vi "INST_PS_MEAS_2.0.0.vi"(4 "Use OPC?(T)":bool=TRUE, 6 "Instrument Select (Output 1)":string(combo)="1", 7 "Clear Error in":bool, 8 "error in (no error)":errorcluster, 9 "Measurement Type (Voltage)":string(combo)="MEAS:VOLT?", 11 "VISA session":refnum<visa-resource-name>) -> (0 "error out":errorcluster, 1 "Measurement (str)":string, 2 "Measurement":dbl format="%.2p", 3 "dup VISA session":refnum<visa-resource-name>)   [LabVIEW 2018]
doc: "This VI takes a measurement on the output signal and returns the measured value."
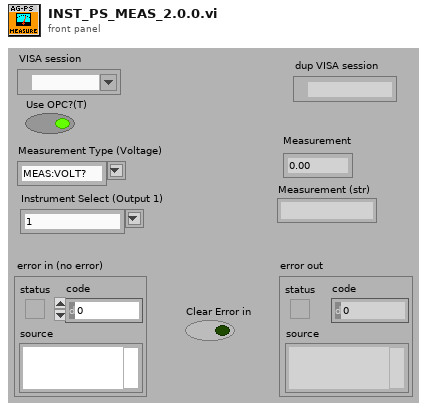
[diagram p1: front panel]
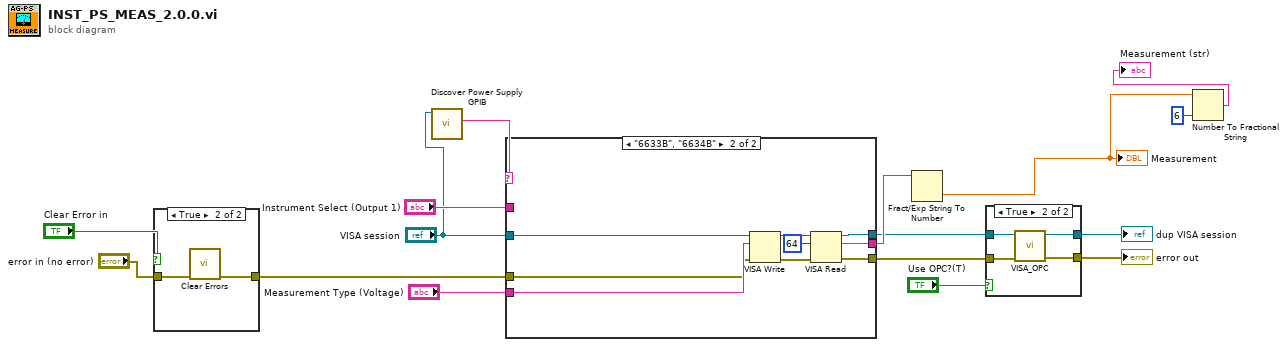
[diagram p0: block diagram]
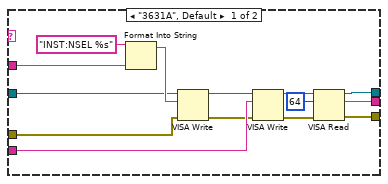
[diagram p2: hidden frame]
diagram:
  n1 = case shown="True" "Clear Error in" {
    tunnel: "error in (no error)" -> [w17 w19]
    tunnel: [w17 w18] -> w7
    frame False {
    }
    frame True {
      n2 = call <vilib>:"Clear Errors.vi"("error in (no error)"=w19) -> ("error out"=w18:errorcluster)  [unwired: 5 in, 1 out]
    }
  }
  n3 = call "Discover Power Supply GPIB.vi"("ADDRESS IN"="VISA session") -> ("PSn Model"=w5:string)  [unwired: 10 in]
  n4 = case shown="\"6633B\", \"6634B\"" w5 {
    tunnel: [w31 w40] -> w16
    tunnel: "Measurement Type (Voltage)" -> [w29 w38]
    tunnel: "Instrument Select (Output 1)" -> [w28 _]
    tunnel: "VISA session" -> [w23 w35]
    tunnel: [w22 w37] -> w13
    tunnel: [w21 w36] -> w10
    tunnel: w7 -> [w20 w34]
    frame "3631A", Default {
      n5 = Format Into String(format string="INST:NSEL %s", w28) -> (resulting string=w26:string)  [unwired: 2 in, 1 out]
      n6 = VISA Write(VISA resource name=w23, write buffer=w26, error in (no error)=w20) -> (VISA resource name out=w24:refnum<visa-resource-name>, error out=w25:errorcluster)  [unwired: 1 out]
      n7 = VISA Write(VISA resource name=w24, write buffer=w29, error in (no error)=w25) -> (VISA resource name out=w30:refnum<visa-resource-name>, error out=w33:errorcluster)  [unwired: 1 out]
      n8 = VISA Read(VISA resource name=w30, byte count=u32 64, error in (no error)=w33) -> (VISA resource name out=w21:refnum<visa-resource-name>, read buffer=w31:string, error out=w22:errorcluster)  [unwired: 1 out]
    }
    frame "6633B", "6634B" {
      n9 = VISA Write(VISA resource name=w35, write buffer=w38, error in (no error)=w34) -> (VISA resource name out=w39:refnum<visa-resource-name>, error out=w42:errorcluster)  [unwired: 1 out]
      n10 = VISA Read(VISA resource name=w39, byte count=u32 64, error in (no error)=w42) -> (VISA resource name out=w36:refnum<visa-resource-name>, read buffer=w40:string, error out=w37:errorcluster)  [unwired: 1 out]
    }
  }
  n11 = Fract/Exp String To Number(string=w16) -> (number=w3:dbl)  [unwired: 3 in, 1 out]
  "Measurement" <- w3
  n12 = case shown="True" "Use OPC?(T)" {
    tunnel: w13 -> [w43 w48]
    tunnel: [w43 w47] -> w12
    tunnel: [w44 w46] -> w11
    tunnel: w10 -> [w44 w45]
    frame False {
    }
    frame True {
      n13 = call "VISA_OPC.vi"("error in"=w48, "Session In"=w45) -> ("error out"=w47:errorcluster, "Session Out"=w46:refnum<visa-resource-name>)  [unwired: 7 in, 1 out]
    }
  }
  "error out" <- w12
  "dup VISA session" <- w11
  n14 = Number To Fractional String(number=w3, precision (6)=i16 6) -> (F-format string=→"Measurement (str)":string)  [unwired: 2 in]
